vi "cRIO_8maze_controls_v2.vi"() -> ()   [LabVIEW 2019]
panel:
  out "Direction array":bool[](array[boolean])=[TRUE, FALSE, FALSE, TRUE, FALSE, TRUE, TRUE, FALSE, TRUE, FALSE, FALSE, TRUE, FALSE, TRUE, FALSE, FALSE, TRUE, FALSE, TRUE, TRUE, FALSE, TRUE, FALSE, FALSE, TRUE, FALSE, TRUE, TRUE, FALSE, TRUE, FALSE, FALSE, TRUE, FALSE, TRUE, TRUE, FALSE, TRUE, FALSE, FALSE, TRUE, FALSE, TRUE, TRUE, FALSE, TRUE, FALSE, FALSE, TRUE]
  out "Seq update":i32
  out "Loop seq.":dbl
  out "Loop seq. R":dbl
  out "All BBR":bool
  out "BB3_R":bool
  out "BB2_R":bool
  out "BB1_R":bool
  out "All BBL":bool
  out "BB3_L":bool
  out "BB2_L":bool
  out "BB1_L":bool
  in  "Num same \nturns in a row":dbl=2.0 format="%#_13g"
  out "Right":bool=TRUE
  out "Loop seq. L":dbl
  in  "Sound":bool
  in  "AIR_R":bool
  in  "AIR_L":bool
  out "Left":bool=TRUE
  in  "MD_R":bool
  in  "MD_L":bool
  in  "LED_R":bool
  in  "LED_L":bool
  in  "PWM rate":dbl[](array[numeric])=[0.1, 0.1, 0.1, 0.1]
  out "appended array":bool[](array[boolean])
  in  "PWM positions":dbl[](array[numeric])=[4.0, 4.4, 8.2, 9.5]
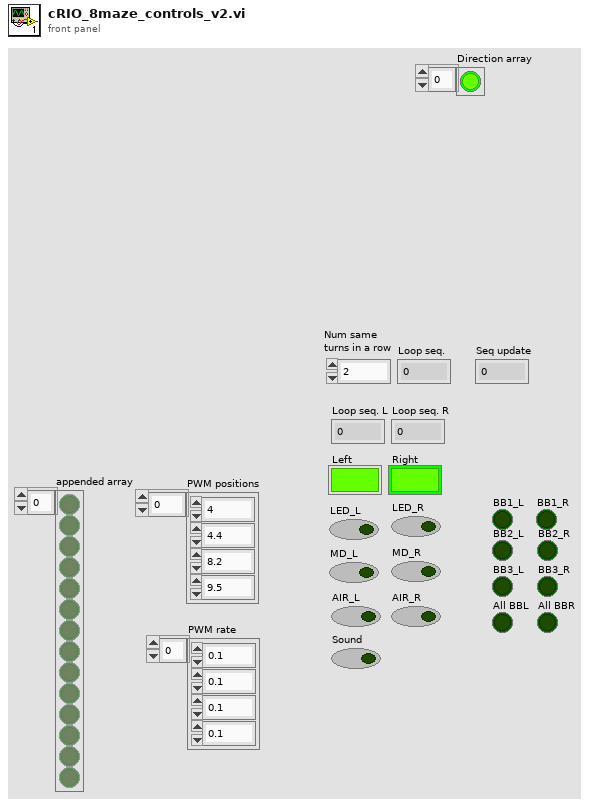
[diagram p1: front panel]
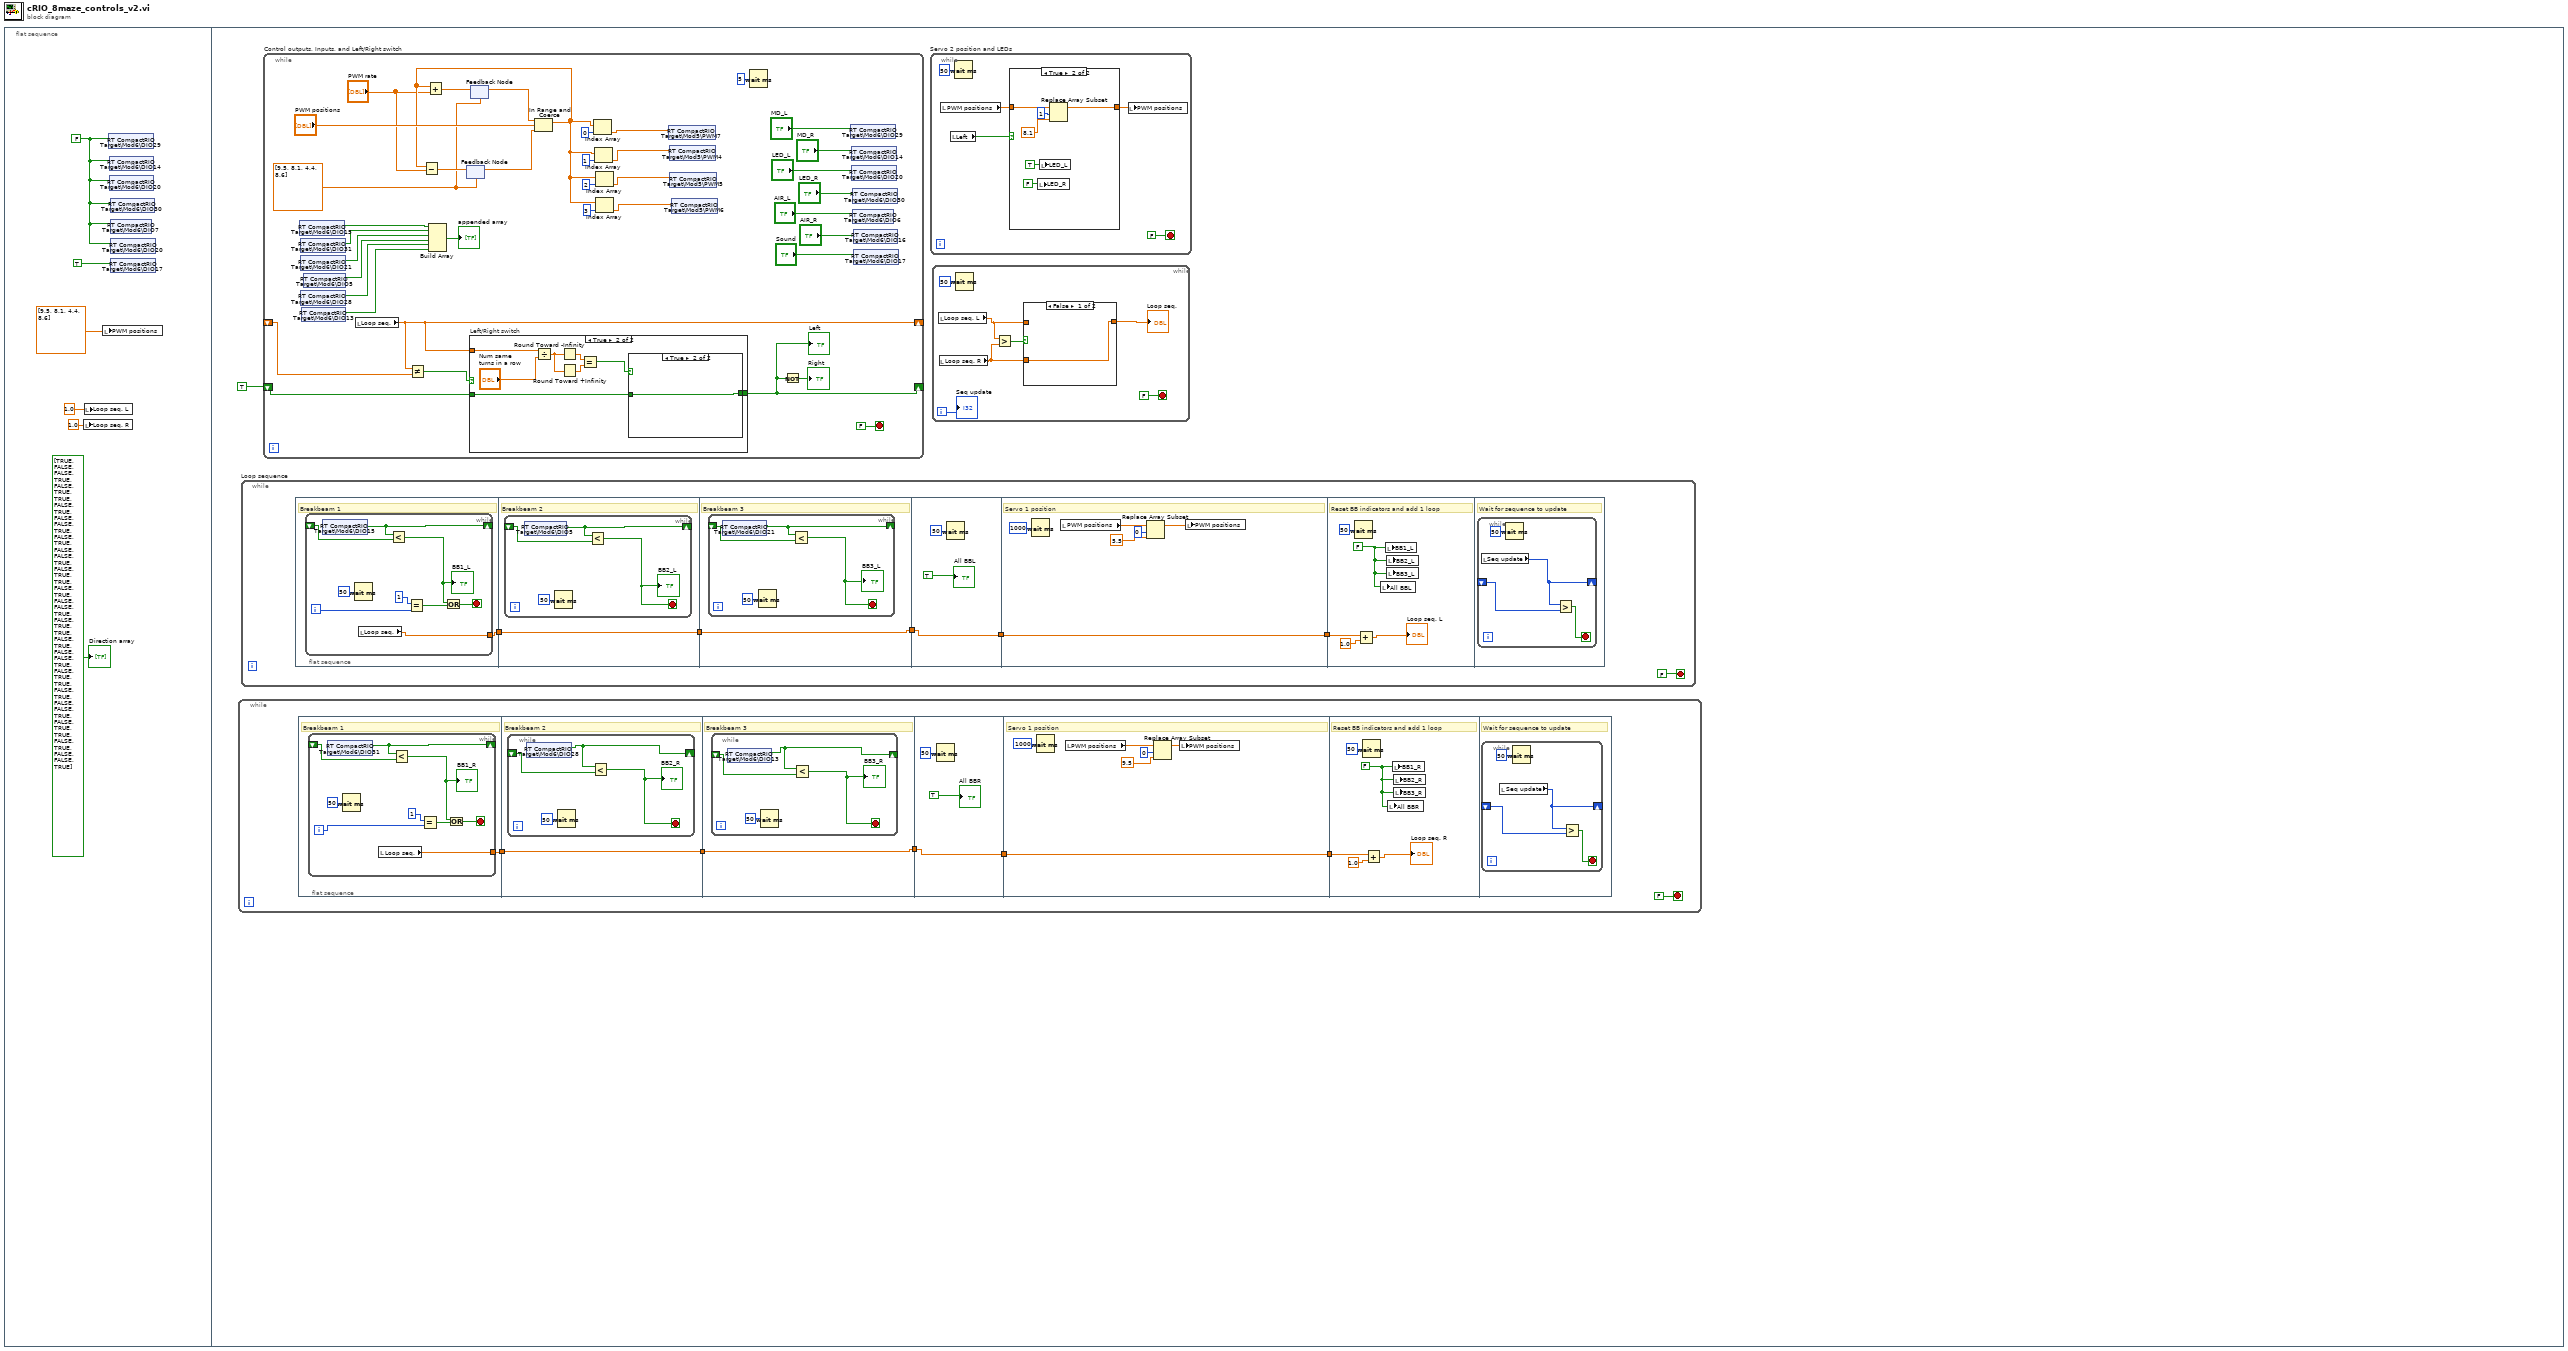
[diagram p0: block diagram]
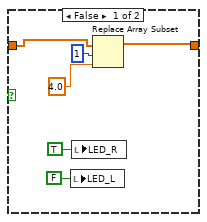
[diagram p3: hidden frame]
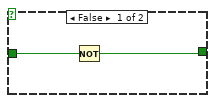
[diagram p5: hidden frame]
diagram:
  n1 = flat-sequence {
    frame #0 {
      w6 = FALSE
      n2 = local write "Loop seq. R"(1.0 ("Loop seq. R")) -> ()
      n3 = local write "Loop seq. L"(1.0 ("Loop seq.")) -> ()
      n4 = local write "PWM positions"(dbl[] [9.5, 8.1, 4.4, 8.6]) -> ()
      n5 = shared-variable "RT CompactRIO Target\\Mod6\\DIO29"(w6) -> ()  [unwired: 1 in, 1 out]
      n6 = shared-variable "RT CompactRIO Target\\Mod6\\DIO14"(w6) -> ()  [unwired: 1 in, 1 out]
      n7 = shared-variable "RT CompactRIO Target\\Mod6\\DIO20"(w6) -> ()  [unwired: 1 in, 1 out]
      n8 = shared-variable "RT CompactRIO Target\\Mod6\\DIO30"(w6) -> ()  [unwired: 1 in, 1 out]
      n9 = shared-variable "RT CompactRIO Target\\Mod6\\DIO7"(w6) -> ()  [unwired: 1 in, 1 out]
      n10 = shared-variable "RT CompactRIO Target\\Mod6\\DIO20"(w6) -> ()  [unwired: 1 in, 1 out]
      n11 = shared-variable "RT CompactRIO Target\\Mod6\\DIO17"(TRUE) -> ()  [unwired: 1 in, 1 out]
      "Direction array" <- bool[] [TRUE, FALSE, FALSE, TRUE, FALSE, TRUE, TRUE, FALSE, TRUE, FALSE, FALSE, TRUE, FALSE, TRUE, FALSE, FALSE, TRUE, FALSE, TRUE, TRUE, FALSE, TRUE, FALSE, FALSE, TRUE, FALSE, TRUE, TRUE, FALSE, TRUE, FALSE, FALSE, TRUE, FALSE, TRUE, TRUE, FALSE, TRUE, FALSE, FALSE, TRUE, FALSE, TRUE, TRUE, FALSE, TRUE, FALSE, FALSE, TRUE]
    }
    frame #1 {
      n12 = while {
        stop <- FALSE stop-if-true
        n13 = flat-sequence {
          tunnel: [w23] -> w21
          tunnel: [w33] -> w20
          tunnel: w21 -> [w33]
          tunnel: [w38] -> w19
          tunnel: w20 -> [w38]
          tunnel: w19 -> [w44]
          tunnel: [w44] -> w18
          tunnel: w18 -> [w51]
          tunnel: [w51] -> w17
          tunnel: w17 -> [w54]
          frame #0 {
            # "Breakbeam 1"
            n14 = while {
              shift-right: [w31] -> _
              shift-left: _ -> [w32]
              tunnel: [w24] -> w23
              i -> [w26]
              stop <- w29 stop-if-true
              n15 = shared-variable "RT CompactRIO Target\\Mod6\\DIO31"() -> (w31:bool)  [unwired: 1 in, 1 out]
              n16 = Wait (ms)(milliseconds to wait=u32 50) -> ()  [unwired: 1 out]
              n17 = local read "Loop seq."() -> (w24:dbl)
              n18 = Less?(x=w31, y=w32) -> (x < y?=w28:bool)
              "BB1_R" <- w28
              n19 = Equal?(x=1, y=w26) -> (x = y?=w25:bool)
              n20 = Or(x=w28, y=w25) -> (x .or. y?=w29:bool)
            }
          }
          frame #1 {
            # "Breakbeam 2"
            n21 = while {
              shift-right: [w35] -> _
              shift-left: _ -> [w37]
              stop <- w34 stop-if-true
              n22 = shared-variable "RT CompactRIO Target\\Mod6\\DIO28"() -> (w35:bool)  [unwired: 1 in, 1 out]
              n23 = Wait (ms)(milliseconds to wait=u32 50) -> ()  [unwired: 1 out]
              n24 = Less?(x=w35, y=w37) -> (x < y?=w34:bool)
              "BB2_R" <- w34
            }
          }
          frame #2 {
            # "Breakbeam 3"
            n25 = while {
              shift-right: [w40] -> _
              shift-left: _ -> [w42]
              stop <- w39 stop-if-true
              n26 = shared-variable "RT CompactRIO Target\\Mod6\\DIO13"() -> (w40:bool)  [unwired: 1 in, 1 out]
              n27 = Wait (ms)(milliseconds to wait=u32 50) -> ()  [unwired: 1 out]
              n28 = Less?(x=w40, y=w42) -> (x < y?=w39:bool)
              "BB3_R" <- w39
            }
          }
          frame #3 {
            n29 = Wait (ms)(milliseconds to wait=u32 50) -> ()  [unwired: 1 out]
            "All BBR" <- TRUE
          }
          frame #4 {
            # "Servo 1 position"
            n30 = Wait (ms)(milliseconds to wait=u32 1000) -> ()  [unwired: 1 out]
            n31 = local read "PWM positions"() -> (w47:dbl[])
            n32 = Replace Array Subset(array=w47, new element=9.5 ("new element/subarray"), index=0) -> (w46:dbl[])
            n33 = local write "PWM positions"(w46) -> ()
          }
          frame #5 {
            w53 = FALSE
            # "Reset BB indicators and add 1 loop"
            n34 = Wait (ms)(milliseconds to wait=u32 50) -> ()  [unwired: 1 out]
            n35 = Add(x=w54, y=1.0) -> (x+y=→"Loop seq. R":dbl)
            n36 = local write "All BBR"(w53) -> ()
            n37 = local write "BB1_R"(w53) -> ()
            n38 = local write "BB2_R"(w53) -> ()
            n39 = local write "BB3_R"(w53) -> ()
          }
          frame #6 {
            # "Wait for sequence to update"
            n40 = while {
              shift-right: [w57] -> _
              shift-left: _ -> [w59]
              stop <- w58 stop-if-true
              n41 = local read "Seq update"() -> (w57:i32)
              n42 = Wait (ms)(milliseconds to wait=u32 50) -> ()  [unwired: 1 out]
              n43 = Greater?(x=w57, y=w59) -> (0:w58:bool)
            }
          }
        }
      }
      n44 = while "Loop sequence" {
        stop <- FALSE stop-if-true
        n45 = flat-sequence {
          tunnel: [w84] -> w82
          tunnel: [w94] -> w83
          tunnel: w82 -> [w94]
          tunnel: [w99] -> w80
          tunnel: w83 -> [w99]
          tunnel: w80 -> [w106]
          tunnel: [w106] -> w79
          tunnel: w79 -> [w112]
          tunnel: [w112] -> w78
          tunnel: w78 -> [w115]
          frame #0 {
            # "Breakbeam 1"
            n46 = while {
              shift-right: [w89] -> _
              shift-left: _ -> [w93]
              tunnel: [w85] -> w84
              i -> [w86]
              stop <- w91 stop-if-true
              n47 = shared-variable "RT CompactRIO Target\\Mod6\\DIO15"() -> (w89:bool)  [unwired: 1 in, 1 out]
              n48 = Wait (ms)(milliseconds to wait=u32 50) -> ()  [unwired: 1 out]
              n49 = local read "Loop seq."() -> (w85:dbl)
              n50 = Less?(x=w89, y=w93) -> (x < y?=w90:bool)
              "BB1_L" <- w90
              n51 = Equal?(x=1, y=w86) -> (x = y?=w87:bool)
              n52 = Or(x=w90, y=w87) -> (x .or. y?=w91:bool)
            }
          }
          frame #1 {
            # "Breakbeam 2"
            n53 = while {
              shift-right: [w96] -> _
              shift-left: _ -> [w98]
              stop <- w95 stop-if-true
              n54 = shared-variable "RT CompactRIO Target\\Mod6\\DIO5"() -> (w96:bool)  [unwired: 1 in, 1 out]
              n55 = Wait (ms)(milliseconds to wait=u32 50) -> ()  [unwired: 1 out]
              n56 = Less?(x=w96, y=w98) -> (x < y?=w95:bool)
              "BB2_L" <- w95
            }
          }
          frame #2 {
            # "Breakbeam 3"
            n57 = while {
              shift-right: [w101] -> _
              shift-left: _ -> [w103]
              stop <- w100 stop-if-true
              n58 = shared-variable "RT CompactRIO Target\\Mod6\\DIO21"() -> (w101:bool)  [unwired: 1 in, 1 out]
              n59 = Wait (ms)(milliseconds to wait=u32 50) -> ()  [unwired: 1 out]
              n60 = Less?(x=w101, y=w103) -> (x < y?=w100:bool)
              "BB3_L" <- w100
            }
          }
          frame #3 {
            n61 = Wait (ms)(milliseconds to wait=u32 50) -> ()  [unwired: 1 out]
            "All BBL" <- TRUE
          }
          frame #4 {
            # "Servo 1 position"
            n62 = Wait (ms)(milliseconds to wait=u32 1000) -> ()  [unwired: 1 out]
            n63 = local read "PWM positions"() -> (w110:dbl[])
            n64 = Replace Array Subset(array=w110, new element=5.5 ("new element/subarray"), index=0) -> (w107:dbl[])
            n65 = local write "PWM positions"(w107) -> ()
          }
          frame #5 {
            w114 = FALSE
            # "Reset BB indicators and add 1 loop"
            n66 = Wait (ms)(milliseconds to wait=u32 50) -> ()  [unwired: 1 out]
            n67 = Add(x=w115, y=1.0) -> (x+y=→"Loop seq. L":dbl)
            n68 = local write "All BBL"(w114) -> ()
            n69 = local write "BB1_L"(w114) -> ()
            n70 = local write "BB2_L"(w114) -> ()
            n71 = local write "BB3_L"(w114) -> ()
          }
          frame #6 {
            # "Wait for sequence to update"
            n72 = while {
              shift-right: [w118] -> _
              shift-left: _ -> [w120]
              stop <- w119 stop-if-true
              n73 = local read "Seq update"() -> (w118:i32)
              n74 = Wait (ms)(milliseconds to wait=u32 50) -> ()  [unwired: 1 out]
              n75 = Greater?(x=w118, y=w120) -> (0:w119:bool)
            }
          }
        }
      }
      n76 = while "Control outputs, Inputs, and Left/Right switch" {
        shift-right: [w127] -> _
        shift-left: TRUE -> [w129]
        shift-right: [w125] -> _
        shift-left: _ -> [w126]
        stop <- FALSE stop-if-true
        w145 = dbl[] [9.5, 8.1, 4.4, 8.6]
        n77 = shared-variable "RT CompactRIO Target\\Mod6\\DIO15"() -> (w139:bool)  [unwired: 1 in, 1 out]
        n78 = shared-variable "RT CompactRIO Target\\Mod6\\DIO31"() -> (w133:bool)  [unwired: 1 in, 1 out]
        n79 = shared-variable "RT CompactRIO Target\\Mod6\\DIO21"() -> (w134:bool)  [unwired: 1 in, 1 out]
        n80 = shared-variable "RT CompactRIO Target\\Mod6\\DIO28"() -> (w136:bool)  [unwired: 1 in, 1 out]
        n81 = shared-variable "RT CompactRIO Target\\Mod6\\DIO13"() -> (w137:bool)  [unwired: 1 in, 1 out]
        n82 = shared-variable "RT CompactRIO Target\\Mod6\\DIO5"() -> (w135:bool)  [unwired: 1 in, 1 out]
        n83 = local read "Loop seq."() -> (w125:dbl)
        n84 = Not Equal?(x=w125, y=w126) -> (x != y?=w124:bool)
        n85 = Build Array(w139, w133, w134, w135, w136, w137) -> (→"appended array":bool[])
        n86 = feedback #1(w145) -> (w146:dbl[])
        n87 = case "Left/Right switch" shown="True" w124 {
          tunnel: w125 -> [_ w168]
          tunnel: w129 -> [w160 w162]
          tunnel: [w160 w161] -> w127
          frame False {
          }
          frame True {
            n88 = Divide(x=w168, y="Num same \nturns in a row") -> (x/y=w166:dbl)
            n89 = Round Toward -Infinity(1:w166) -> (0:w165:dbl)
            n90 = Round Toward +Infinity(x=w166) -> (ceil(x): smallest int >= x=w164:dbl)
            n91 = Equal?(x=w165, y=w164) -> (x = y?=w163:bool)
            n92 = case shown="True" w163 {
              tunnel: [w169 w171] -> w161
              tunnel: w162 -> [w170 w171]
              frame False {
                n93 = Not(x=w170) -> (.not. x?=w169:bool)
              }
              frame True {
              }
            }
          }
        }
        "Left" <- w127
        n94 = feedback #2(w145) -> (w149:dbl[])
        n95 = In Range and Coerce(upper limit=w149, x="PWM positions", lower limit=w146) -> (coerced(x)=w148:dbl[])  [unwired: 1 out]
        n96 = Subtract(x=w148, y="PWM rate") -> (x-y=w147:dbl[])
        n97 = Add(x=w148, y="PWM rate") -> (x+y=w150:dbl[])
        n98 = feedback-in #1(w147) -> ()
        n99 = feedback-in #2(w150) -> ()
        n100 = Index Array(array=w148, index=0) -> (element=w123:dbl)
        n101 = Index Array(array=w148, index=1) -> (element=w122:dbl)
        n102 = Index Array(array=w148, index=2) -> (element=w158:dbl)
        n103 = Index Array(array=w148, index=3) -> (element=w159:dbl)
        n104 = shared-variable "RT CompactRIO Target\\Mod5\\PWM7"(w123) -> ()  [unwired: 1 in, 1 out]
        n105 = shared-variable "RT CompactRIO Target\\Mod5\\PWM4"(w122) -> ()  [unwired: 1 in, 1 out]
        n106 = shared-variable "RT CompactRIO Target\\Mod5\\PWM5"(w158) -> ()  [unwired: 1 in, 1 out]
        n107 = shared-variable "RT CompactRIO Target\\Mod5\\PWM6"(w159) -> ()  [unwired: 1 in, 1 out]
        n108 = Wait (ms)(milliseconds to wait=u32 5) -> ()  [unwired: 1 out]
        n109 = Not(x=w127) -> (.not. x?=→"Right":bool)
        n110 = shared-variable "RT CompactRIO Target\\Mod6\\DIO29"("MD_L") -> ()  [unwired: 1 in, 1 out]
        n111 = shared-variable "RT CompactRIO Target\\Mod6\\DIO14"("MD_R") -> ()  [unwired: 1 in, 1 out]
        n112 = shared-variable "RT CompactRIO Target\\Mod6\\DIO20"("LED_L") -> ()  [unwired: 1 in, 1 out]
        n113 = shared-variable "RT CompactRIO Target\\Mod6\\DIO30"("LED_R") -> ()  [unwired: 1 in, 1 out]
        n114 = shared-variable "RT CompactRIO Target\\Mod6\\DIO6"("AIR_L") -> ()  [unwired: 1 in, 1 out]
        n115 = shared-variable "RT CompactRIO Target\\Mod6\\DIO16"("AIR_R") -> ()  [unwired: 1 in, 1 out]
        n116 = shared-variable "RT CompactRIO Target\\Mod6\\DIO17"("Sound") -> ()  [unwired: 1 in, 1 out]
      }
      n117 = while "Servo 2 position and LEDs" {
        stop <- FALSE stop-if-true
        n118 = local read "PWM positions"() -> (w63:dbl[])
        n119 = local read "Left"() -> (w64:bool)
        n120 = Wait (ms)(milliseconds to wait=u32 50) -> ()  [unwired: 1 out]
        n121 = case shown="True" w64 {
          tunnel: w63 -> [w69 w75]
          tunnel: [w68 w74] -> w62
          frame False {
            n122 = local write "LED_L"(FALSE ("LED_L")) -> ()
            n123 = local write "LED_R"(TRUE ("LED_R")) -> ()
            n124 = Replace Array Subset(array=w69, new element=4.0 ("new element/subarray"), index=1) -> (w68:dbl[])
          }
          frame True {
            n125 = local write "LED_R"(FALSE ("LED_R")) -> ()
            n126 = local write "LED_L"(TRUE ("LED_L")) -> ()
            n127 = Replace Array Subset(array=w75, new element=8.1 ("new element/subarray"), index=1) -> (w74:dbl[])
          }
        }
        n128 = local write "PWM positions"(w62) -> ()
      }
      n129 = while {
        i -> [w8]
        stop <- FALSE stop-if-true
        n130 = local read "Loop seq. L"() -> (w13:dbl)
        n131 = local read "Loop seq. R"() -> (w12:dbl)
        n132 = Wait (ms)(milliseconds to wait=u32 50) -> ()  [unwired: 1 out]
        n133 = Greater?(x=w13, y=w12) -> (0:w14:bool)
        n134 = case shown="False" w14 {
          tunnel: [w15 w16] -> w11
          tunnel: w13 -> [_ w16]
          tunnel: w12 -> [w15 _]
          frame False {
          }
          frame True {
          }
        }
        "Loop seq." <- w11
        "Seq update" <- w8
      }
    }
  }
